vi "frontEnd.vi"(8 "error in (no error)":errorcluster, 11 "PixelflySettings in":refnum<class "PixelflySettings.lvclass">) -> (0 "error out":errorcluster, 3 "PixelflySettings out":refnum<class "PixelflySettings.lvclass">)   [LabVIEW 2011, in "Tools.lvlib" / "Settings.lvlib" / "PixelflySettings.lvclass"]
uses:
  PixelflySettings.lvclass
  PixelflySettings.lvclass/PixelflySettings.ctl
  Settings.lvlib
panel:
  in  "Camera":enum16{"Pixis", "ProEM", "PixelFly"}(ring)
  in  "Save Images":bool
  in  "Save as":bool
  out "Path":path
  in  "Mode":enum16{"Asynch Shutter", "Double Shot", "Video"}(ring)=enum."Double Shot"
  in  "Vertical Binning":enum16{"1", "2"}(ring)
  in  "Horizonatal Binning":enum16{"1", "2"}(ring)
  in  "image_number":i32 caption="Image Number"
  in  "Close":bool
  in  "Open":bool
  in  "Save":bool
  in  "Triggering":bool
  in  "gain":enum16{"Low", "High"}(ring) caption="Gain"
  in  "exposure":dbl(slide)=0.0064 min=1e-05 max=10.0 step=1e-05 scale=1e-05..0.01 scale format="%^#_6g"
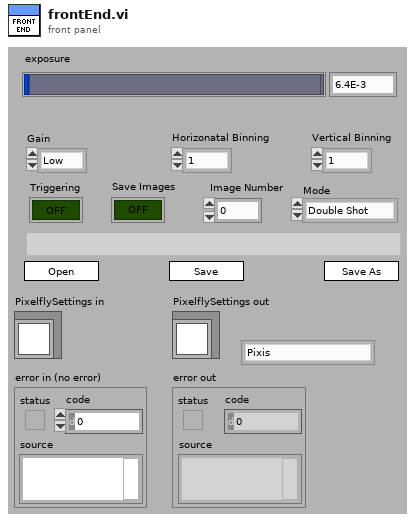
[diagram p1: front panel]
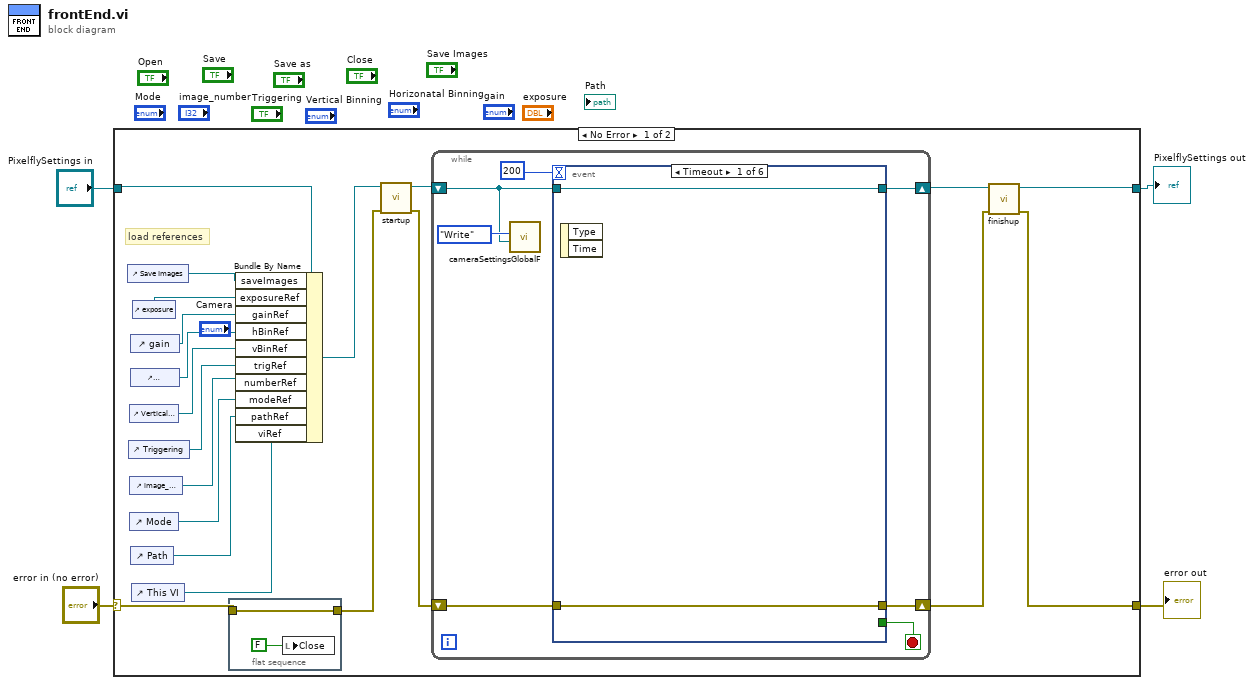
[diagram p0: block diagram]
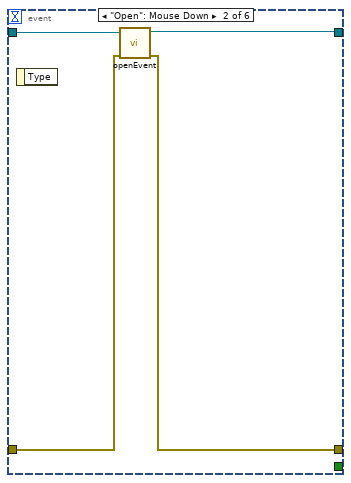
[diagram p2: hidden frame]
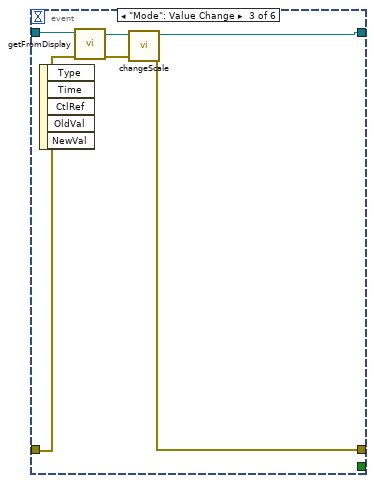
[diagram p3: hidden frame]
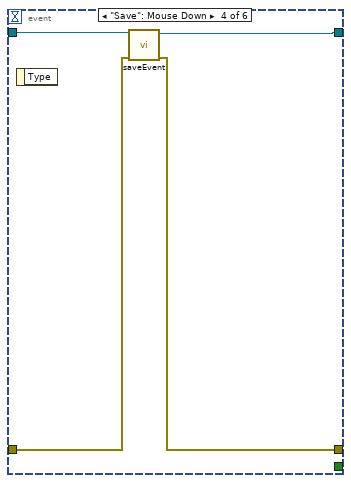
[diagram p4: hidden frame]
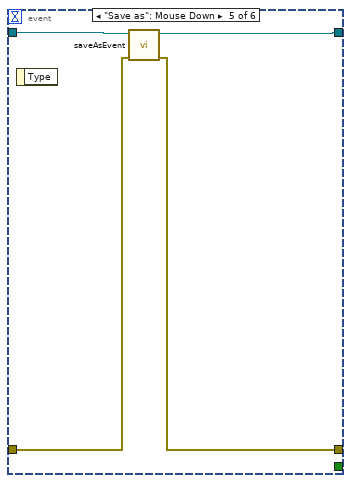
[diagram p5: hidden frame]
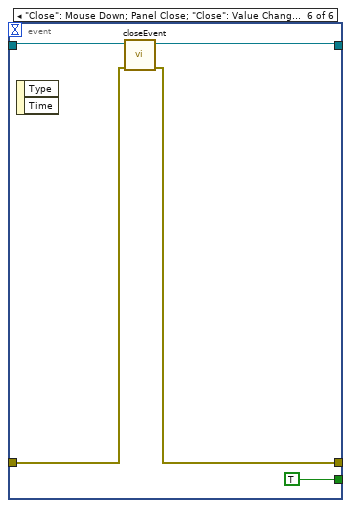
[diagram p6: hidden frame]
diagram:
  n1 = case shown="No Error" "error in (no error)" {
    selector: "error in (no error)" -> [w7 w59]
    tunnel: [w19 w59] -> w3
    tunnel: [w21 w60] -> w2
    tunnel: "PixelflySettings in" -> [w12 w60]
    frame No Error {
      # "load references"
      n2 = control-ref of="Save Images"() -> (w5:refnum<vi>)
      n3 = control-ref of="Triggering"() -> (w14:refnum<vi>)
      n4 = control-ref of="Vertical Binning"() -> (w15:refnum<vi>)
      n5 = control-ref of="image_number"() -> (w13:refnum<vi>)
      n6 = control-ref of="Mode"() -> (w8:refnum<vi>)
      n7 = control-ref of="gain"() -> (w17:refnum<vi>)
      n8 = control-ref of="Horizonatal Binning"() -> (w16:refnum<vi>)
      n9 = control-ref of="Path"() -> (w10:refnum<vi>)
      n10 = control-ref of="This VI"() -> (w9:refnum<vi>)
      n11 = control-ref of="exposure"() -> (w18:refnum<vi>)
      n12 = flat-sequence {
        tunnel: w7 -> [w25]
        tunnel: [w25] -> w6
        frame #0 {
          n13 = local write "Close"(FALSE) -> ()
        }
      }
      n14 = Bundle By Name(cluster=w12, "saveImages"=w5, "exposureRef"=w18, "gainRef"=w17, "hBinRef"=w16, "vBinRef"=w15, "trigRef"=w14, "numberRef"=w13, "modeRef"=w8, "pathRef"=w10, "viRef"=w9) -> (w11:refnum<class "PixelflySettings.lvclass">)
      n15 = call "startup.vi"("error in (no error)"=w6, "PixelflySettings in"=w11) -> ("error out"=w23:errorcluster, "PixelflySettings out"=w24:refnum<class "PixelflySettings.lvclass">)  [unwired: 8 in]
      n16 = while {
        shift-right: [w33] -> w22
        shift-left: w24 -> [w28]
        shift-right: [w32] -> w20
        shift-left: w23 -> [w31]
        stop <- w30 stop-if-true
        n17 = call "cameraSettingsGlobalF.vi"("CamaraSettings"=w28, "Action"=enum16{"Write", "Read"}."Write") -> ()  [unwired: 9 in, 1 out]
        n18 = event shown="[0] Timeout" {
          selector: _ -> [_ _ _ _ _ _]
          dyn-events: _ -> [_ _ _ _ _ _]
          timeout: 200 -> [_ _ _ _ _ _]
          tunnel: [w35 w38 w45 w48 w52 w56] -> w33
          tunnel: w28 -> [w35 w39 w42 w49 w53 w57]
          tunnel: [w34 w36 w44 w46 w50 w54] -> w32
          tunnel: w31 -> [w34 w37 w40 w47 w51 w55]
          tunnel: [_ _ _ _ _ TRUE] -> w30
          event Timeout {
            n19 = event-data() -> ()  [unwired: 1 in, 2 out]
          }
          event "Open": Mouse Down {
            n20 = event-data() -> ()  [unwired: 1 in, 1 out]
            n21 = call "openEvent.vi"("error in (no error)"=w37, "PixelflySettings in"=w39) -> ("error out"=w36:errorcluster, "PixelflySettings out"=w38:refnum<class "PixelflySettings.lvclass">)  [unwired: 8 in]
          }
          event "Mode": Value Change {
            n22 = event-data() -> ()  [unwired: 1 in, 5 out]
            n23 = call "getFromDisplay.vi"("error in (no error)"=w40, "PixelflySettings in"=w42) -> ("error out"=w41:errorcluster, "PixelflySettings out"=w43:refnum<class "PixelflySettings.lvclass">)  [unwired: 8 in]
            n24 = call "changeScale.vi"("error in (no error)"=w41, "PixelflySettings in"=w43) -> ("error out"=w44:errorcluster, "PixelflySettings out"=w45:refnum<class "PixelflySettings.lvclass">)  [unwired: 8 in]
          }
          event "Save": Mouse Down {
            n25 = event-data() -> ()  [unwired: 1 in, 1 out]
            n26 = call "saveEvent.vi"("error in (no error)"=w47, "PixelflySettings in"=w49) -> ("error out"=w46:errorcluster, "PixelflySettings out"=w48:refnum<class "PixelflySettings.lvclass">)  [unwired: 8 in]
          }
          event "Save as": Mouse Down {
            n27 = event-data() -> ()  [unwired: 1 in, 1 out]
            n28 = call "saveAsEvent.vi"("error in (no error)"=w51, "PixelflySettings in"=w53) -> ("error out"=w50:errorcluster, "PixelflySettings out"=w52:refnum<class "PixelflySettings.lvclass">)  [unwired: 8 in]
          }
          event "Close": Mouse Down; Panel Close; "Close": Value Change {
            n29 = event-data() -> ()  [unwired: 1 in, 2 out]
            n30 = call "closeEvent.vi"("error in (no error)"=w55, "PixelflySettings in"=w57) -> ("error out"=w54:errorcluster, "PixelflySettings out"=w56:refnum<class "PixelflySettings.lvclass">)  [unwired: 8 in]
          }
        }
      }
      n31 = call "finishup.vi"("error in (no error)"=w20, "PixelflySettings in"=w22) -> ("error out"=w19:errorcluster, "PixelflySettings out"=w21:refnum<class "PixelflySettings.lvclass">)  [unwired: 8 in]
    }
    frame Error {
    }
  }
  "error out" <- w3
  "PixelflySettings out" <- w2
